vi "DHE_DRV_open_driver.vi"(0 "devno":i32, 11 "error in (no error)":errorcluster) -> (4 "refnum":i32, 15 "error out":errorcluster)   [LabVIEW 2016]
doc: "This VI passes the addressing information in the instrument decriptor to the Instr Open VI and returns the instrument ID. You can optionally reset the instrument by setting the front panel reset control. You must run this VI before using any of the instrument driver VIs for this instrument."
uses:
  c/lib/libarcDHE.so
panel:
  in  "err":i32
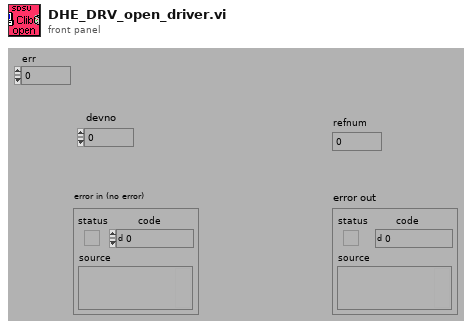
[diagram p1: front panel]
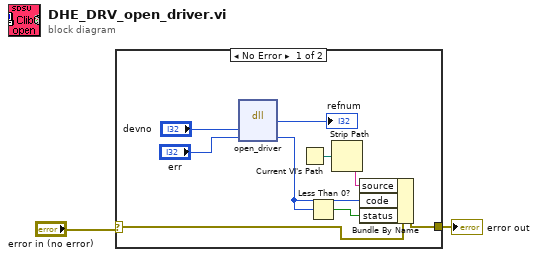
[diagram p0: block diagram]
diagram:
  n1 = case shown="No Error" "error in (no error)" {
    selector: "error in (no error)" -> [w6 w12]
    tunnel: [w9 w12] -> w2
    frame No Error {
      n2 = dll-call lib="home/simager/panview/PAN/Modules/SDSU/private/c/lib/libarcDHE.so" fn="open_driver"("device"="devno", "err"="err") -> ("return type"=→"refnum":i32, "err"=w4:i32)  [unwired: 4 in, 2 out]
      n3 = Current VI's Path() -> (path=w11:path)
      n4 = Less Than 0?(x=w4) -> (x < 0?=w8:bool)
      n5 = Strip Path(path=w11) -> (name=w7:string)  [unwired: 1 out]
      n6 = Bundle By Name(cluster=w6, "source"=w7, "code"=w4, "status"=w8) -> (w9:errorcluster)
    }
    frame Error {
    }
  }
  "error out" <- w2
